vi "_script_fix_Parse State Queue in Find Parse State Queue vi name.vi"   [LabVIEW 2014]
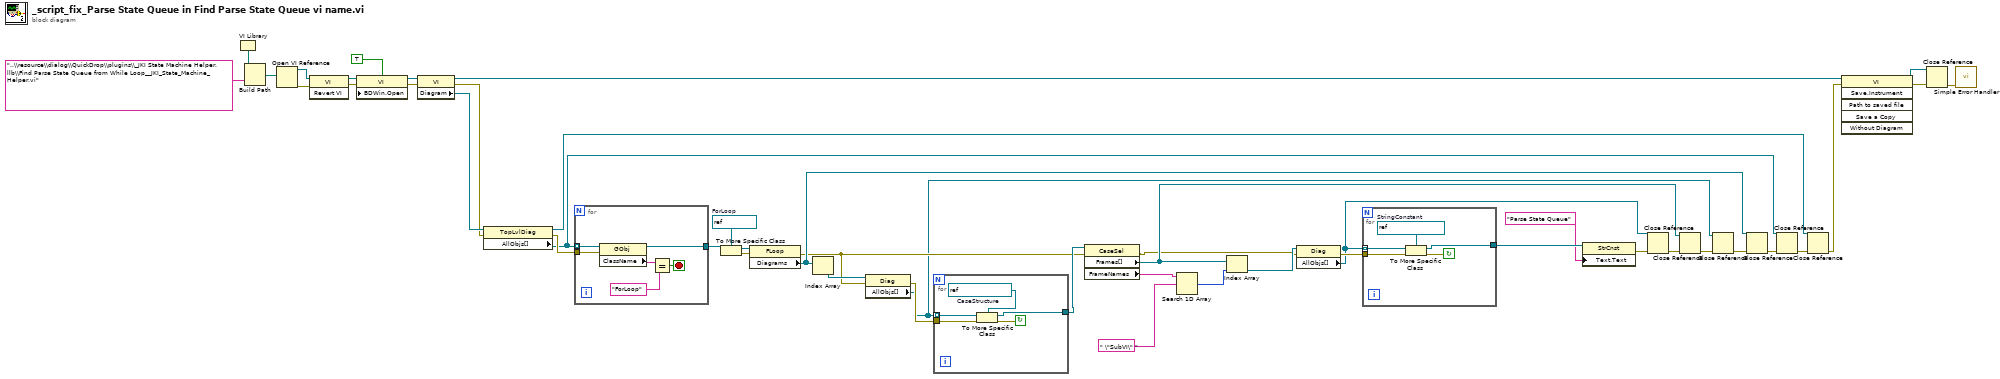
[diagram p0: block diagram]
diagram:
  w33 = refnum<vi> refnum  # ForLoop
  n1 = VI Library() -> (path=w44:path)
  n2 = Build Path(base path=w44, name or relative path="..\\resource\\dialog\\QuickDrop\\plugins\\_JKI State Machine Helper.llb\\Find Parse State Queue from While Loop__JKI_State_Machine_Helper.vi") -> (appended path=w42:path)
  n3 = Open VI Reference(vi path=w42) -> (vi reference=w45:refnum<vi>, error out=w46:errorcluster)  [unwired: 5 in]
  n4 = invoke class="VI" method="Revert VI"(reference=w45, error in=w46) -> (reference out=w20:refnum<vi>, error out=w19:errorcluster)  [unwired: 1 in, 1 out]
  n5 = property class="VI"(reference=w20, error in=w19, "BDWin.Open"=TRUE ("Block Diagram Window:Open")) -> (reference out=w18:refnum<vi>, error out=w17:errorcluster)
  n6 = property class="VI"(reference=w18, error in=w17) -> (reference out=w41:refnum<vi>, error out=w36:errorcluster, "Diagram"=w37:refnum<vi>)
  n7 = property class="TopLvlDiag"(reference=w37, error in=w36) -> (reference out=w22:refnum<vi>, error out=w35:errorcluster, "AllObjs[]"=w24:refnum<vi>[])
  n8 = for {
    tunnel: w24 -> [w52] mode=indexing
    tunnel: w35 -> [w51]
    tunnel: [w50] -> w34
    stop <- w47 stop-if-true
    n9 = property class="GObj"(reference=w52, error in=w51) -> (reference out=w50:refnum<vi>, "ClassName"=w49:string)  [unwired: 1 out]
    n10 = Equal?(x=w49, y="ForLoop") -> (x = y?=w47:bool)
  }
  n11 = To More Specific Class(target class=w33, reference=w34) -> (specific class reference=w32:refnum<vi>, error out=w31:errorcluster)  [unwired: 1 in]
  n12 = property class="FLoop"(reference=w32, error in=w31) -> (error out=w11:errorcluster, "Diagrams"=w15:refnum<vi>[])  [unwired: 1 out]
  n13 = Index Array(array=w15) -> (element=w14:refnum<vi>)  [unwired: 1 in]
  n14 = property class="Diag"(reference=w14, error in=w11) -> (error out=w13:errorcluster, "AllObjs[]"=w7:refnum<vi>[])  [unwired: 1 out]
  n15 = for {
    tunnel: w7 -> [w57] mode=indexing
    tunnel: w13 -> [w56]
    tunnel: [w54] -> w12
    stop <- w55 continue-if-true
    w53 = refnum<vi> refnum  # CaseStructure
    n16 = To More Specific Class(target class=w53, reference=w57, error in=w56) -> (specific class reference=w54:refnum<vi>, error out=w55:errorcluster)
  }
  n17 = property class="CaseSel"(reference=w12, error in=w11) -> (error out=w1:errorcluster, "Frames[]"=w4:refnum<vi>[], "FrameNames"=w6:string[])  [unwired: 1 out]
  n18 = Search 1D Array(1D array=w6, element=" \"SubVI\" " ("y")) -> (index of element=w3:i32)  [unwired: 1 in]
  n19 = Index Array(array=w4, index=w3) -> (element=w2:refnum<vi>)
  n20 = property class="Diag"(reference=w2, error in=w1) -> (error out=w30:errorcluster, "AllObjs[]"=w26:refnum<vi>[])  [unwired: 1 out]
  n21 = for {
    tunnel: w26 -> [w62] mode=indexing
    tunnel: w30 -> [w61]
    tunnel: [w58] -> w29
    stop <- w59 continue-if-true
    w60 = refnum<vi> refnum  # StringConstant
    n22 = To More Specific Class(target class=w60, reference=w62, error in=w61) -> (specific class reference=w58:refnum<vi>, error out=w59:errorcluster)
  }
  n23 = property class="StrCnst"(reference=w29, "Text.Text"="Parse State Queue") -> (error out=w27:errorcluster)  [unwired: 1 in, 1 out]
  n24 = Close Reference(reference=w26, error in (no error)=w27) -> (error out=w10:errorcluster)
  n25 = Close Reference(reference=w4, error in (no error)=w10) -> (error out=w9:errorcluster)
  n26 = Close Reference(reference=w7, error in (no error)=w9) -> (error out=w8:errorcluster)
  n27 = Close Reference(reference=w15, error in (no error)=w8) -> (error out=w25:errorcluster)
  n28 = Close Reference(reference=w24, error in (no error)=w25) -> (error out=w23:errorcluster)
  n29 = Close Reference(reference=w22, error in (no error)=w23) -> (error out=w21:errorcluster)
  n30 = invoke class="VI" method="Save.Instrument"(reference=w41, error in=w21) -> (reference out=w39:refnum<vi>, error out=w40:errorcluster)  [unwired: 4 in, 4 out]
  n31 = Close Reference(reference=w39, error in (no error)=w40) -> (error out=w38:errorcluster)
  n32 = call <vilib>:"Simple Error Handler.vi"("error in (no error)"=w38) -> ()  [unwired: 4 in, 5 out]
